vi "set Period.vi"(10 "Period [s]":dbl, 11 "Timer in":refnum<class "Timer.lvclass">) -> (3 "Timer out":refnum<class "Timer.lvclass">)   [LabVIEW 2015, in "Timer.lvclass"]
uses:
  Timer.lvclass
  Timer.lvclass/Timer.ctl
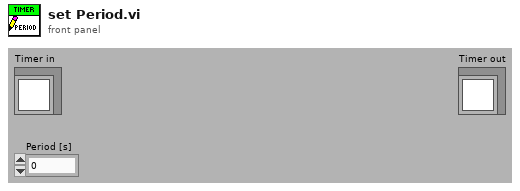
[diagram p1: front panel]
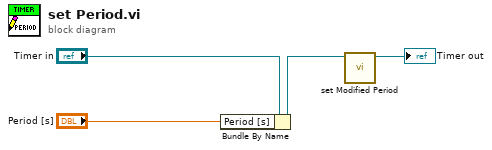
[diagram p0: block diagram]
diagram:
  n1 = Bundle By Name(cluster="Timer in", "Period [s]"="Period [s]") -> (w2:refnum<class "Timer.lvclass">)
  n2 = call "set Modified Period.vi"("Timer in"=w2) -> ("Timer out"=→"Timer out":refnum<class "Timer.lvclass">)  [unwired: 10 in]
